vi "BIO_should_retry.vi"(8 "error in (no error)":errorcluster, 11 "BIO in":refnum<class "BIO.lvclass">) -> (0 "error out":errorcluster, 2 "Should retry":bool, 3 "BIO out":refnum<class "BIO.lvclass">)   [LabVIEW 2013, in "SSL_Lib.lvlib" / "BIO.lvclass"]
uses:
  BIO.lvclass
  SSL-Lib/SSL-Lib.lvclass/SSL-Lib.ctl
  BIO.lvclass/BIO.ctl
  SSL-Lib/Read Crypto Library Path.vi
  Read Handle.vi
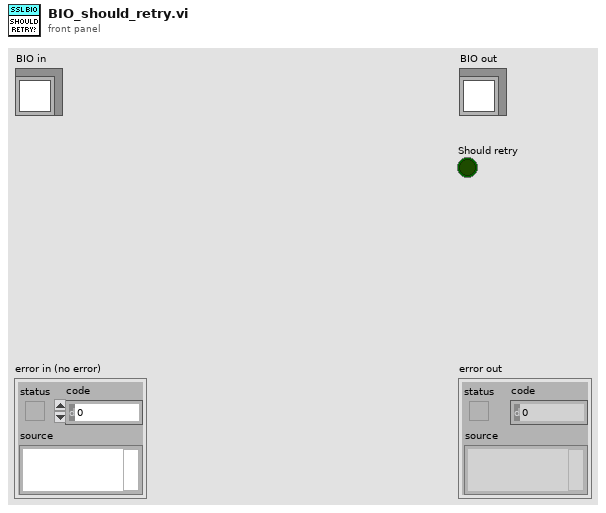
[diagram p1: front panel]
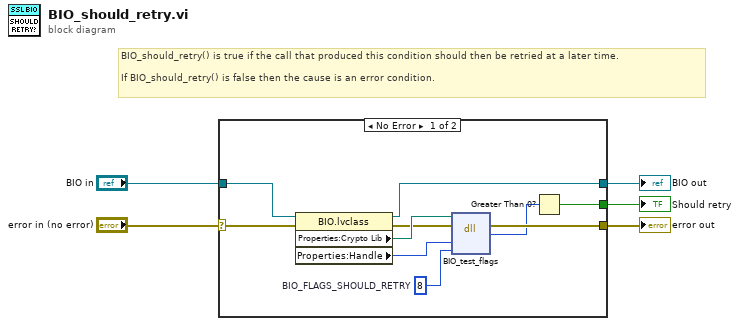
[diagram p0: block diagram]
diagram:
  # "BIO_should_retry() is true if the call that produced this condition should then be retried at a later time.\n\nIf BIO_should_retry() is false then the cause is an error condition."
  n1 = case shown="No Error" "error in (no error)" {
    selector: "error in (no error)" -> [w15 w17]
    tunnel: [w8 w17] -> w4
    tunnel: [w9 w16] -> w2
    tunnel: "BIO in" -> [w12 w16]
    tunnel: [w6 _] -> w1
    frame No Error {
      w10 = 8  # BIO_FLAGS_SHOULD_RETRY
      n2 = property class="BIO.lvclass"(reference=w12, error in=w15) -> (reference out=w9:refnum<class "BIO.lvclass">, error out=w11:errorcluster, "Properties:Crypto Lib"=w13:path, "Properties:Handle"=w14:u64)
      n3 = dll-call lib="C:/Program Files (x86)/National Instruments/Shared/nissl/NIlibeay32.dll" fn="BIO_test_flags"(path in=w13, error in=w11, "BIO"=w14, "flag"=w10) -> (error out=w8:errorcluster, "return type"=w7:i32)  [unwired: 3 in, 1 out]
      n4 = Greater Than 0?(x=w7) -> (x > 0?=w6:bool)
    }
    frame Error {
    }
  }
  "error out" <- w4
  "BIO out" <- w2
  "Should retry" <- w1
